vi "get Name.vi"(11 "Hardware.lvlib:CCD.lvlib:CCD Configuration.lvclass":refnum<class "CCD Configuration.lvclass">) -> (2 "Category string":string, 3 "reference out":refnum<class "CCD Configuration.lvclass">)   [LabVIEW 2016, in "CCD.lvlib" / "CCD Configuration.lvclass"]
uses:
  <userlib>/Common Components/Hardware/CCD/CCD Configuration.lvclass
  <userlib>/Common Components/Hardware/CCD/CCD Configuration.lvclass/CCD Configuration.ctl
  <userlib>/Common Components/Hardware/Abstract Hardware/Hardware.lvclass/Hardware.ctl
  <userlib>/Common Components/Hardware/CCD/CCD Configuration/Read Hardware.lvlib_CCD.lvlib_CCD.lvclass.vi
  <userlib>/Common Components/Hardware/Abstract Hardware/Read Label.vi
  <userlib>/Common Components/Hardware/CCD/CCD/CCD.lvclass
  C:/Program Files (x86)/National Instruments/LabVIEW 2016/user.lib/Common Components/Hardware/Abstract Hardware/Hardware.lvclass
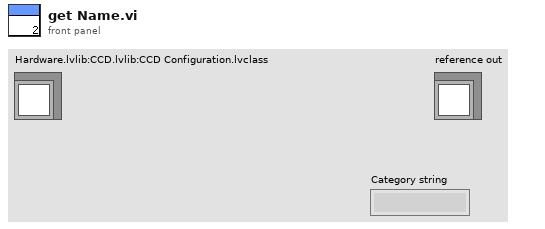
[diagram p1: front panel]
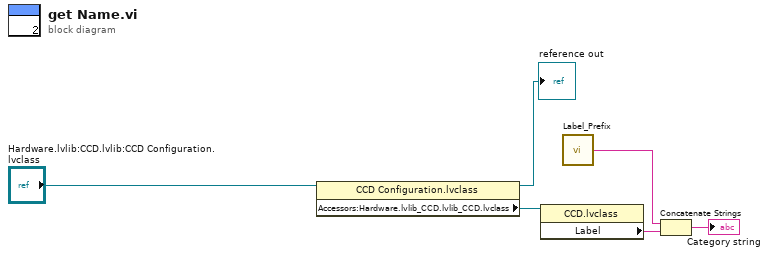
[diagram p0: block diagram]
diagram:
  n1 = property class="CCD Configuration.lvclass"(reference="Hardware.lvlib:CCD.lvlib:CCD Configuration.lvclass") -> (reference out=→"reference out":refnum<class "CCD Configuration.lvclass">, "Accessors:Hardware.lvlib_CCD.lvlib_CCD.lvclass"=w4:refnum<class "CCD.lvclass">)  [unwired: 1 in, 1 out]
  n2 = property class="CCD.lvclass"(reference=w4) -> ("Label"=w5:string)  [unwired: 1 in, 2 out]
  n3 = call <userlib>:"Label_Prefix.vi"() -> ("Label Prefix String"=w3:string)
  n4 = Concatenate Strings(w3, w5) -> (→"Category string":string)
